vi "LiDAR_UI.vi"() -> ()   [LabVIEW 2020]
doc: "This template is for the Queued Message Handler design pattern.\n\nThe Event Handling Loop generates messages based on user interface actions.\n\nThe Message Handling Loop processes messages generated by the Event Handling Loop, or by other messages. The messages are string values, so new messages can be added easily to the Message Cases case structure in the Message Handling Loop. Each message cluster can also provide an optional value for Message Data, which is a variant that can be converted to whatever message-specific data is required."
uses:
  controls/UI Data.ctl
  support/Message Queue/Enqueue Message (Single).vi
  <vilib>/Instr/_visa.llb/VISA Configure Serial Port (Instr).vi
  <vilib>/Utility/error.llb/Error Cluster From Error Code.vi
  <vilib>/ErrorRing/Error Ring.xnode
  support/Message Queue/Message Queue.lvlib
  support/User Event - Stop/User Event - Stop.lvlib
  <vilib>/Analysis/NI_AALBase.lvlib
panel:
  in  "?":T1(tab)
  out "Waveform Graph":dbl[](graph)
  in  "LASER ON/OFF":bool
  out "Duty Cycle":dbl(slide) scale=0.0..0.001
  in  "Exit":bool
  in  "Pulse Length (ns)":dbl(slide) scale=8.0..100.0
  in  "Rep. Rate (Hz)":dbl(slide) scale=0.0..100.0
  in  "Save Settings\nPLCS":bool
  in  "Load Settings\nPLCS":bool
  out "Power (mW)":dbl(slide) scale=0.0..65.0
  out "Warning":bool
  in  "Calibration Current":dbl
  in  "Driver Voltage":dbl
  in  "Save Settings BFS":bool
  in  "TEC Current Limit (A)":dbl(slide) scale=0.0..1.0
  in  "TEC KI":dbl(slide) scale=0.0..0.04
  in  "TEC KP":dbl(slide) scale=0.0..2.0
  in  "TEC Temperatur":dbl(knob) scale=0.0..70.0
  in  "VREF (V)":dbl(slide) scale=0.0..1.0
  in  "Load Settings BFS":bool
  out "Display (BFS-VRM 03)":string
  in  "Numeric":dbl
  in  "Un/Lock":bool
  out "Display (PLCS-21/LDP-V)":string
  in  "Set Max. Duty Cycle":dbl
  in  "Voltage (mv)":dbl(slide) scale=0.0..5600.0
  in  "Current (mA)":u64(slide) scale=0.0..10.0
  in  "Modes":enum32{"Voltage Mode", "Current Mode"}(radio)
  # "Pulser Parameter"
  # "Toggles"
  # "Warnings"
  # "Driver Parameter"
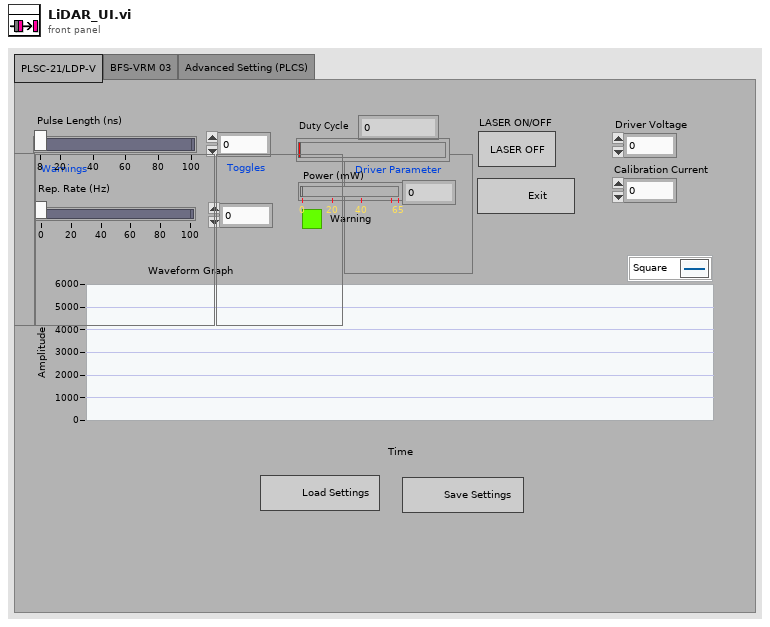
[diagram p1: front panel]
types:
  T1 = enum32{"PLSC-21/LDP-V", "BFS-VRM 03", "Advanced Setting (PLCS)"}
  T2 = typedef "UI Data.ctl" = cluster{"Boolean <Replace Me>":bool, "String <Replace Me>":string, "Numeric <Replace Me>":dbl, "LASER ON/OFF Ref":refnum<vi>, "Do Something Else Ref":refnum<vi>, "Data Display Ref":refnum<vi>, "Exit Button Ref":refnum<vi>}
  T3 = typedef "Message Queue.lvlib/All Message Queues.ctl" = cluster{"UI":refnum<queue>}
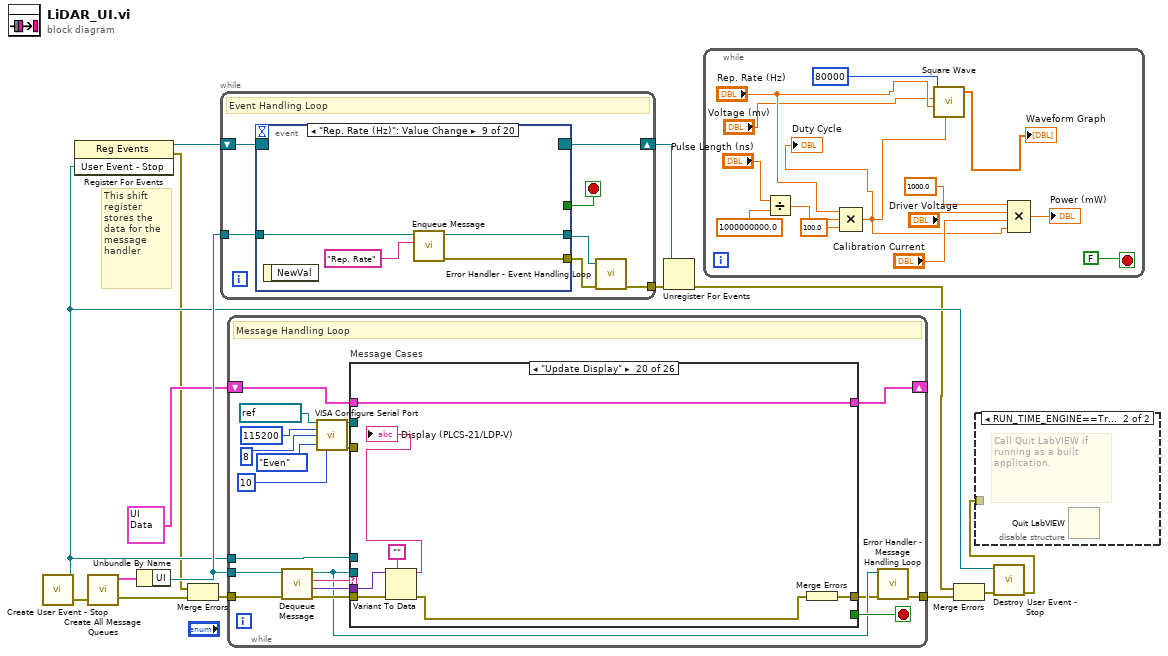
[diagram p0: block diagram]
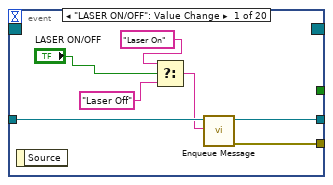
[diagram p3: hidden frame]
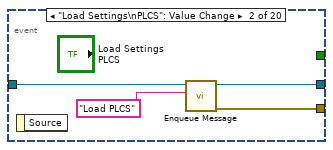
[diagram p4: hidden frame]
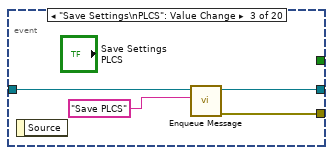
[diagram p5: hidden frame]
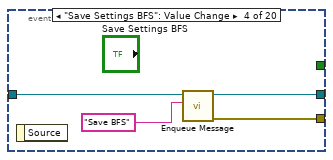
[diagram p6: hidden frame]
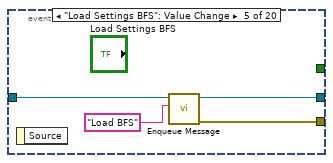
[diagram p7: hidden frame]
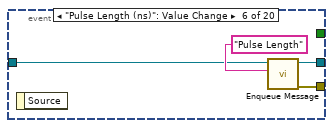
[diagram p8: hidden frame]
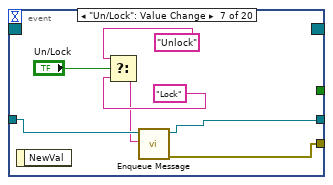
[diagram p9: hidden frame]
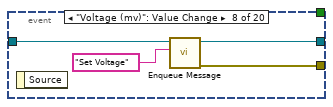
[diagram p10: hidden frame]
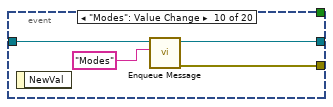
[diagram p11: hidden frame]
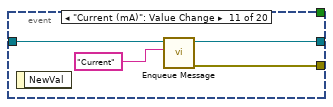
[diagram p12: hidden frame]
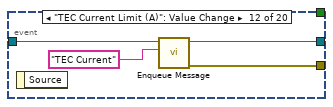
[diagram p13: hidden frame]
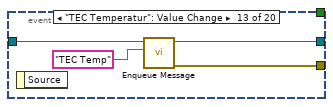
[diagram p14: hidden frame]
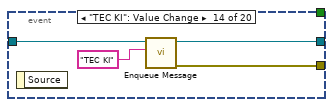
[diagram p15: hidden frame]
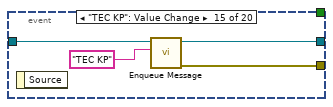
[diagram p16: hidden frame]
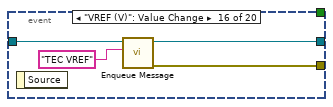
[diagram p17: hidden frame]
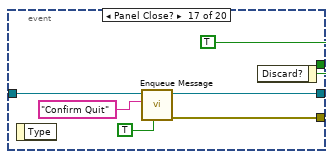
[diagram p18: hidden frame]
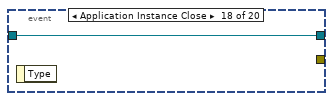
[diagram p19: hidden frame]
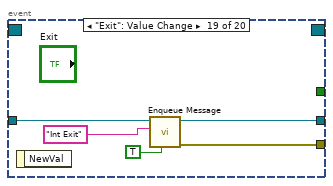
[diagram p20: hidden frame]
diagram:
  # "This shift register stores the data for the message handler"
  n1 = call "Create User Event - Stop.vi"() -> ("error out"=w11:errorcluster, "User Event - Stop"=w5:refnum<user-event>)  [unwired: 10 in]
  n2 = register-events(w5) -> (reference out=w6:refnum<event-registration>, error out=w3:errorcluster)  [unwired: 2 in]
  n3 = call "Create All Message Queues.vi"("error in (no error)"=w11) -> ("error out"=w15:errorcluster, "Message Queues out"=w14:T3)  [unwired: 9 in]
  n4 = Unbundle By Name(w14) -> ("UI"=w12:refnum<queue>)
  n5 = Merge Errors(w3, w15) -> (w4:errorcluster)
  n6 = while {
    tunnel: w12 -> [w22]
    shift-right: [w17] -> w9
    shift-left: w6 -> [w21]
    tunnel: [w19] -> w7
    stop <- w16 stop-if-true
    # "Event Handling Loop"
    n7 = event shown="[8] \"Rep. Rate (Hz)\": Value Change" {
      selector: w21 -> [_ _ _ _ _ _ _ _ _ _ _ _ _ _ _ _ _ _ _ _]
      dyn-events: [_ _ _ _ _ _ _ _ _ _ _ _ _ _ _ _ _ _ _ _] -> w17
      timeout: _ -> [_ _ _ _ _ _ _ _ _ _ _ _ _ _ _ _ _ _ _ _]
      tunnel: [_ _ _ _ _ _ _ _ _ _ _ _ _ _ _ _ _ _ _ TRUE ("Discard?")] -> w16
      tunnel: w22 -> [w29 w33 w37 w40 w44 w46 w54 w60 w64 w68 w72 w76 w80 w84 w88 w92 w97 w99 w104 w107]
      tunnel: [w27 w30 w34 w38 w42 w47 w53 w58 w61 w65 w70 w73 w77 w81 w85 w89 w96 _ w103 _] -> w20
      tunnel: [w28 w32 w36 w41 w45 w48 w55 w59 w63 w67 w71 w75 w79 w83 w87 w91 w95 w99 w102 w107] -> w18
      event "LASER ON/OFF": Value Change {
        n8 = event-data() -> ()  [unwired: 1 in, 1 out]
        n9 = Select(t="Laser On" ("Message"), s="LASER ON/OFF", f="Laser Off" ("Message")) -> (s? t:f=w26:string)
        n10 = call-poly "Enqueue Message.vi"("Message"=w26, "Message Queue"=w29) -> ("error out"=w27:errorcluster, "dup Message Queue"=w28:refnum<queue>)  [unwired: 8 in]
      }
      event "Load Settings\nPLCS": Value Change {
        n11 = event-data() -> ()  [unwired: 1 in, 1 out]
        n12 = call-poly "Enqueue Message.vi"("Message"="Load PLCS", "Message Queue"=w33) -> ("error out"=w30:errorcluster, "dup Message Queue"=w32:refnum<queue>)  [unwired: 8 in]
      }
      event "Save Settings\nPLCS": Value Change {
        n13 = event-data() -> ()  [unwired: 1 in, 1 out]
        n14 = call-poly "Enqueue Message.vi"("Message"="Save PLCS", "Message Queue"=w37) -> ("error out"=w34:errorcluster, "dup Message Queue"=w36:refnum<queue>)  [unwired: 8 in]
      }
      event "Save Settings BFS": Value Change {
        n15 = event-data() -> ()  [unwired: 1 in, 1 out]
        n16 = call-poly "Enqueue Message.vi"("Message"="Save BFS", "Message Queue"=w40) -> ("error out"=w38:errorcluster, "dup Message Queue"=w41:refnum<queue>)  [unwired: 8 in]
      }
      event "Load Settings BFS": Value Change {
        n17 = event-data() -> ()  [unwired: 1 in, 1 out]
        n18 = call-poly "Enqueue Message.vi"("Message"="Load BFS", "Message Queue"=w44) -> ("error out"=w42:errorcluster, "dup Message Queue"=w45:refnum<queue>)  [unwired: 8 in]
      }
      event "Pulse Length (ns)": Value Change {
        n19 = event-data() -> ()  [unwired: 1 in, 1 out]
        n20 = call-poly "Enqueue Message.vi"("Message"="Pulse Length", "Message Queue"=w46) -> ("error out"=w47:errorcluster, "dup Message Queue"=w48:refnum<queue>)  [unwired: 8 in]
      }
      event "Un/Lock": Value Change {
        n21 = event-data() -> ()  [unwired: 1 in, 1 out]
        n22 = Select(t="Unlock", s="Un/Lock", f="Lock") -> (s? t:f=w50:string)
        n23 = call-poly "Enqueue Message.vi"("Message"=w50, "Message Queue"=w54) -> ("error out"=w53:errorcluster, "dup Message Queue"=w55:refnum<queue>)  [unwired: 8 in]
      }
      event "Voltage (mv)": Value Change {
        n24 = event-data() -> ()  [unwired: 1 in, 1 out]
        n25 = call-poly "Enqueue Message.vi"("Message"="Set Voltage", "Message Queue"=w60) -> ("error out"=w58:errorcluster, "dup Message Queue"=w59:refnum<queue>)  [unwired: 8 in]
      }
      event "Rep. Rate (Hz)": Value Change {
        n26 = event-data() -> ()  [unwired: 1 in, 1 out]
        n27 = call-poly "Enqueue Message.vi"("Message"="Rep. Rate", "Message Queue"=w64) -> ("error out"=w61:errorcluster, "dup Message Queue"=w63:refnum<queue>)  [unwired: 8 in]
      }
      event "Modes": Value Change {
        n28 = event-data() -> ()  [unwired: 1 in, 1 out]
        n29 = call-poly "Enqueue Message.vi"("Message"="Modes", "Message Queue"=w68) -> ("error out"=w65:errorcluster, "dup Message Queue"=w67:refnum<queue>)  [unwired: 8 in]
      }
      event "Current (mA)": Value Change {
        n30 = event-data() -> ()  [unwired: 1 in, 1 out]
        n31 = call-poly "Enqueue Message.vi"("Message"="Current", "Message Queue"=w72) -> ("error out"=w70:errorcluster, "dup Message Queue"=w71:refnum<queue>)  [unwired: 8 in]
      }
      event "TEC Current Limit (A)": Value Change {
        n32 = event-data() -> ()  [unwired: 1 in, 1 out]
        n33 = call-poly "Enqueue Message.vi"("Message"="TEC Current", "Message Queue"=w76) -> ("error out"=w73:errorcluster, "dup Message Queue"=w75:refnum<queue>)  [unwired: 8 in]
      }
      event "TEC Temperatur": Value Change {
        n34 = event-data() -> ()  [unwired: 1 in, 1 out]
        n35 = call-poly "Enqueue Message.vi"("Message"="TEC Temp", "Message Queue"=w80) -> ("error out"=w77:errorcluster, "dup Message Queue"=w79:refnum<queue>)  [unwired: 8 in]
      }
      event "TEC KI": Value Change {
        n36 = event-data() -> ()  [unwired: 1 in, 1 out]
        n37 = call-poly "Enqueue Message.vi"("Message"="TEC KI", "Message Queue"=w84) -> ("error out"=w81:errorcluster, "dup Message Queue"=w83:refnum<queue>)  [unwired: 8 in]
      }
      event "TEC KP": Value Change {
        n38 = event-data() -> ()  [unwired: 1 in, 1 out]
        n39 = call-poly "Enqueue Message.vi"("Message"="TEC KP", "Message Queue"=w88) -> ("error out"=w85:errorcluster, "dup Message Queue"=w87:refnum<queue>)  [unwired: 8 in]
      }
      event "VREF (V)": Value Change {
        n40 = event-data() -> ()  [unwired: 1 in, 1 out]
        n41 = call-poly "Enqueue Message.vi"("Message"="TEC VREF", "Message Queue"=w92) -> ("error out"=w89:errorcluster, "dup Message Queue"=w91:refnum<queue>)  [unwired: 8 in]
      }
      event Panel Close? {
        n42 = event-data() -> ()  [unwired: 1 in, 1 out]
        n43 = call-poly "Enqueue Message.vi"("Priority Message? (F)"=TRUE, "Message"="Confirm Quit", "Message Queue"=w97) -> ("error out"=w96:errorcluster, "dup Message Queue"=w95:refnum<queue>)  [unwired: 7 in]
        n44 = event-data("Discard?"=TRUE) -> ()  [unwired: 1 in, 1 out]
      }
      event Application Instance Close {
        n45 = event-data() -> ()  [unwired: 1 in, 1 out]
      }
      event "Exit": Value Change {
        n46 = event-data() -> ()  [unwired: 1 in, 1 out]
        n47 = call-poly "Enqueue Message.vi"("Priority Message? (F)"=TRUE, "Message"="Int Exit", "Message Queue"=w104) -> ("error out"=w103:errorcluster, "dup Message Queue"=w102:refnum<queue>)  [unwired: 7 in]
      }
      event User Event {
        n48 = event-data() -> ()  [unwired: 1 in, 1 out]
        n49 = local write "Display (PLCS-21/LDP-V)"("\"Exit\" button pressed/COM Released" ("VI Stopped")) -> ()
      }
    }
    n50 = call "Error Handler - Event Handling Loop.vi"("error in (no error)"=w20, "Message Queue"=w18) -> ("dup error in"=w19:errorcluster)  [unwired: 8 in, 1 out]
  }
  n51 = while {
    tunnel: w12 -> [w118]
    shift-right: [w125] -> _
    shift-left: T2 {"Boolean <Replace Me>"=FALSE, "String <Replace Me>"="", "Numeric <Replace Me>"=0.0, "LASER ON/OFF Ref"=refnum, "Do Something Else Ref"=refnum, "Data Display Ref"=refnum, "Exit Button Ref"=refnum} ("Data Cluster") -> [w126]
    tunnel: w5 -> [w123]
    tunnel: w4 -> [w122]
    tunnel: [w116] -> w13
    stop <- w124 stop-if-true
    # "Message Handling Loop"
    n52 = call "Dequeue Message.vi"("error in (no error)"=w122, "Message Queue"=w118) -> ("error out"=w121:errorcluster, "Message Data"=w119:variant, "Message"=w120:string, "dup Message Queue"=w117:refnum<queue>)  [unwired: 6 in]
    n53 = call-poly "VISA Configure Serial Port"("VISA resource name"=refnum<visa-resource-name> "COM4", "baud rate (9600)"=u32 115200, "data bits (8)"=u16 8, "parity (0:none)"=enum16{"None", "Odd", "Even", "Mark", "Space"}."Even", "stop bits (10: 1 bit)"=u16 10) -> ("VISA resource name out"=w109:refnum<visa-resource-name>, "error out"=w108:errorcluster)  [unwired: 9 in]
    n54 = case "Message Cases" shown="\"Update Display\"" w120 {
      selector: w120 -> [_ _ _ _ _ _ _ _ _ _ _ _ _ _ _ _ _ _ _ _ _ _ _ _ _ w431]
      tunnel: w117 -> [w134 w153 w168 w186 w205 w211 w236 w254 w272 w290 w308 w319 w330 _ _ _ _ _ _ _ _ _ w401 w408 w430 _]
      tunnel: w121 -> [w135 w154 w170 w188 w207 w213 w238 w256 w274 w292 w310 w321 w332 w342 w345 w353 w361 w369 w377 w383 w389 w398 w405 w409 w423 _]
      tunnel: [w133 w156 w169 w187 w206 w212 w237 w255 w273 w291 w309 w322 w333 w342 w345 w353 w361 w369 w377 w384 w390 w392 w403 w413 w426 w432] -> w115
      tunnel: w126 -> [w140 w143 w173 w179 w210 w222 w240 w258 w276 w294 w312 w323 w334 w341 w344 w352 w360 w368 w376 w378 w391 w397 w404 w414 w429 w433]
      tunnel: [w139 w143 w173 w179 w210 w222 w240 w258 w276 w294 w312 w323 w334 w341 w344 w352 w360 w368 w376 w378 w391 w397 w404 w414 w429 w433] -> w125
      tunnel: [_ _ _ _ _ _ _ _ _ _ _ _ _ _ _ _ _ _ _ _ _ _ _ _ TRUE _] -> w124
      tunnel: w119 -> [_ _ _ _ _ _ _ _ _ _ _ _ _ _ _ _ _ _ _ w382 w388 w396 _ _ w420 _]
      tunnel: w123 -> [_ _ _ _ _ _ _ _ _ _ _ _ _ _ _ _ _ _ _ _ _ _ _ _ w425 _]
      tunnel: w109 -> [_ w161 w172 w194 w204 w221 _ _ _ _ _ w317 w326 _ _ _ _ _ _ _ _ _ _ _ w419 _]
      tunnel: w108 -> [_ w160 w171 w193 w203 w220 _ _ _ _ _ w316 w325 _ _ _ _ _ _ _ _ _ _ _ w418 _]
      frame "Initialize" {
        w132 = "Laser Off" ("Initial Message")
        # "Initialize - All initialization work should take place in this message, since other loops can potentially enqueue messages that execute immediately after this one."
        n55 = control-ref of="Exit"() -> (w137:refnum<vi>)
        n56 = control-ref of="Display (PLCS-21/LDP-V)"() -> (w138:refnum<vi>)
        n57 = control-ref of="LASER ON/OFF"() -> (w136:refnum<vi>)
        n58 = property on="Pulse Length (ns)" class="Slide (strict)"("Scale.Maximum"="Numeric") -> ()  [unwired: 2 in, 2 out]
        n59 = local write "Warning"(FALSE) -> ()
        n60 = call-poly "Enqueue Message.vi"("error in (no error)"=w135, "Message"=w132, "Message Queue"=w134) -> ("error out"=w133:errorcluster)  [unwired: 7 in, 1 out]
        n61 = Bundle By Name(cluster=w140, "LASER ON/OFF Ref"=w136, "Data Display Ref"=w138, "Exit Button Ref"=w137, "String <Replace Me>"=w132) -> (w139:T2)
        n62 = call "Convert to Dynamic Data"("Array"=dbl[] [] ("History Data")) -> ("Dynamic Data Type"=w129:dynamicdata)  [unwired: 3 in]
        n63 = call "Convert from Dynamic Data"("Dynamic Data Type"=w129) -> ("Array"=w127:dbl[])  [unwired: 3 in]
        n64 = local write "Waveform Graph"(w127) -> ()
      }
      frame "Pulse Length" {
        n65 = local read "Pulse Length (ns)"() -> (w155:dbl)
        n66 = local read "Duty Cycle"() -> (w150:dbl)
        n67 = Concatenate Strings("Laseroff" ("Message"), "\r") -> (w144:string)
        n68 = Number To Decimal String(number=w155) -> (decimal integer string=w158:string)  [unwired: 1 in]
        n69 = Greater?(x=w150, y="Set Max. Duty Cycle") -> (0:w141:bool)
        "Warning" <- w141
        n70 = Select(t="Laser Off" ("Message"), s=w141, f="Update Display" ("Message")) -> (s? t:f=w149:string)
        n71 = Concatenate Strings("spulse ", w158, "\r") -> (w152:string)
        n72 = Select(t=w152, s=w141, f=w144) -> (s? t:f=w151:string)
        n73 = VISA Write(VISA resource name=w161, write buffer=w151, error in (no error)=w160) -> ()  [unwired: 3 out]
        n74 = call-poly "Enqueue Message.vi"("error in (no error)"=w154, "Message Data"=w151, "Message"=w149, "Message Queue"=w153) -> ("error out"=w156:errorcluster)  [unwired: 6 in, 1 out]
      }
      frame "Set Voltage" {
        n75 = local read "Voltage (mv)"() -> (w162:dbl)
        n76 = Number To Decimal String(number=w162) -> (decimal integer string=w165:string)  [unwired: 1 in]
        n77 = Concatenate Strings("svoltage  ", w165, "\r") -> (w163:string)
        n78 = VISA Write(VISA resource name=w172, write buffer=w163, error in (no error)=w171) -> ()  [unwired: 3 out]
        n79 = call-poly "Enqueue Message.vi"("error in (no error)"=w170, "Message Data"=w163, "Message"="Update Display", "Message Queue"=w168) -> ("error out"=w169:errorcluster)  [unwired: 6 in, 1 out]
      }
      frame "Rep. Rate" {
        n80 = local read "Set Max. Duty Cycle"() -> (w175:dbl)
        n81 = local read "Rep. Rate (Hz)"() -> (w189:dbl)
        n82 = local read "Duty Cycle"() -> (w180:dbl)
        n83 = Concatenate Strings("laseroff ", "\r") -> (w182:string)
        n84 = Number To Decimal String(number=w189) -> (decimal integer string=w191:string)  [unwired: 1 in]
        n85 = Greater?(x=w180, y=w175) -> (0:w174:bool)
        n86 = Select(t="Laser Off" ("Message"), s=w174, f="Update Display" ("Message")) -> (s? t:f=w177:string)
        n87 = Concatenate Strings("sreprate  ", w191, "\r") -> (w185:string)
        n88 = Select(t=w185, s=w174, f=w182) -> (s? t:f=w181:string)
        n89 = VISA Write(VISA resource name=w194, write buffer=w181, error in (no error)=w193) -> ()  [unwired: 3 out]
        n90 = local write "Warning"(w174) -> ()
        n91 = call-poly "Enqueue Message.vi"("error in (no error)"=w188, "Message Data"=w181, "Message"=w177, "Message Queue"=w186) -> ("error out"=w187:errorcluster)  [unwired: 6 in, 1 out]
      }
      frame "Modes" {
        n92 = Equal To 0?(x="Modes") -> (x = 0?=w209:bool)
        n93 = Select(t=1, s=w209, f=2) -> (s? t:f=w200:i32)
        n94 = Number To Decimal String(number=w200) -> (decimal integer string=w199:string)  [unwired: 1 in]
        n95 = Concatenate Strings("smode ", w199, "\r") -> (w195:string)
        n96 = VISA Write(VISA resource name=w204, write buffer=w195, error in (no error)=w203) -> ()  [unwired: 3 out]
        n97 = call-poly "Enqueue Message.vi"("error in (no error)"=w207, "Message Data"=w195, "Message"="Update Display", "Message Queue"=w205) -> ("error out"=w206:errorcluster)  [unwired: 6 in, 1 out]
      }
      frame "Current" {
        n98 = Number To Decimal String(number="Current (mA)") -> (decimal integer string=w219:string)  [unwired: 1 in]
        n99 = Concatenate Strings("scurrent  ", w219, "\r") -> (w215:string)
        n100 = VISA Write(VISA resource name=w221, write buffer=w215, error in (no error)=w220) -> ()  [unwired: 3 out]
        n101 = call-poly "Enqueue Message.vi"("error in (no error)"=w213, "Message Data"=w215, "Message"="Update Display", "Message Queue"=w211) -> ("error out"=w212:errorcluster)  [unwired: 6 in, 1 out]
      }
      frame "TEC Current" {
        n102 = local read "TEC Current Limit (A)"() -> (w235:dbl)
        n103 = call-poly "VISA Configure Serial Port"("VISA resource name"=refnum<visa-resource-name> "COM3", "baud rate (9600)"=u32 115200, "data bits (8)"=u16 8, "parity (0:none)"=enum16{"None", "Odd", "Even", "Mark", "Space"}."Even", "stop bits (10: 1 bit)"=u16 10) -> ("VISA resource name out"=w224:refnum<visa-resource-name>, "error out"=w223:errorcluster)  [unwired: 9 in]
        n104 = Number To Fractional String(number=w235, precision (6)=2) -> (F-format string=w234:string)  [unwired: 2 in]
        n105 = Concatenate Strings("simax  ", w234, "\r") -> (w230:string)
        n106 = VISA Write(VISA resource name=w224, write buffer=w230, error in (no error)=w223) -> ()  [unwired: 3 out]
        n107 = call-poly "Enqueue Message.vi"("error in (no error)"=w238, "Message Data"=w230, "Message"="Display 2", "Message Queue"=w236) -> ("error out"=w237:errorcluster)  [unwired: 6 in, 1 out]
      }
      frame "TEC Temp" {
        w250 = "stsoll  "  # stsoll
        n108 = local read "TEC Temperatur"() -> (w253:dbl)
        n109 = call-poly "VISA Configure Serial Port"("VISA resource name"=refnum<visa-resource-name> "COM3", "baud rate (9600)"=u32 115200, "data bits (8)"=u16 8, "parity (0:none)"=enum16{"None", "Odd", "Even", "Mark", "Space"}."Even", "stop bits (10: 1 bit)"=u16 10) -> ("VISA resource name out"=w242:refnum<visa-resource-name>, "error out"=w241:errorcluster)  [unwired: 9 in]
        n110 = Number To Fractional String(number=w253, precision (6)=0) -> (F-format string=w252:string)  [unwired: 2 in]
        n111 = Concatenate Strings(w250, w252, "\r") -> (w248:string)
        n112 = VISA Write(VISA resource name=w242, write buffer=w248, error in (no error)=w241) -> ()  [unwired: 3 out]
        n113 = call-poly "Enqueue Message.vi"("error in (no error)"=w256, "Message Data"=w248, "Message"="Display 2", "Message Queue"=w254) -> ("error out"=w255:errorcluster)  [unwired: 6 in, 1 out]
      }
      frame "TEC KI" {
        w268 = "ski  "  # ski
        n114 = local read "TEC KI"() -> (w271:dbl)
        n115 = call-poly "VISA Configure Serial Port"("VISA resource name"=refnum<visa-resource-name> "COM3", "baud rate (9600)"=u32 115200, "data bits (8)"=u16 8, "parity (0:none)"=enum16{"None", "Odd", "Even", "Mark", "Space"}."Even", "stop bits (10: 1 bit)"=u16 10) -> ("VISA resource name out"=w260:refnum<visa-resource-name>, "error out"=w259:errorcluster)  [unwired: 9 in]
        n116 = Number To Fractional String(number=w271, precision (6)=2) -> (F-format string=w270:string)  [unwired: 2 in]
        n117 = Concatenate Strings(w268, w270, "\r") -> (w266:string)
        n118 = VISA Write(VISA resource name=w260, write buffer=w266, error in (no error)=w259) -> ()  [unwired: 3 out]
        n119 = call-poly "Enqueue Message.vi"("error in (no error)"=w274, "Message Data"=w266, "Message"="Display 2", "Message Queue"=w272) -> ("error out"=w273:errorcluster)  [unwired: 6 in, 1 out]
      }
      frame "TEC KP" {
        w286 = "skp  "  # skp
        n120 = local read "TEC KP"() -> (w289:dbl)
        n121 = call-poly "VISA Configure Serial Port"("VISA resource name"=refnum<visa-resource-name> "COM3", "baud rate (9600)"=u32 115200, "data bits (8)"=u16 8, "parity (0:none)"=enum16{"None", "Odd", "Even", "Mark", "Space"}."Even", "stop bits (10: 1 bit)"=u16 10) -> ("VISA resource name out"=w278:refnum<visa-resource-name>, "error out"=w277:errorcluster)  [unwired: 9 in]
        n122 = Number To Fractional String(number=w289, precision (6)=2) -> (F-format string=w288:string)  [unwired: 2 in]
        n123 = Concatenate Strings(w286, w288, "\r") -> (w284:string)
        n124 = VISA Write(VISA resource name=w278, write buffer=w284, error in (no error)=w277) -> ()  [unwired: 3 out]
        n125 = call-poly "Enqueue Message.vi"("error in (no error)"=w292, "Message Data"=w284, "Message"="Display 2", "Message Queue"=w290) -> ("error out"=w291:errorcluster)  [unwired: 6 in, 1 out]
      }
      frame "TEC VREF" {
        w304 = "svref "  # svref
        n126 = local read "VREF (V)"() -> (w307:dbl)
        n127 = call-poly "VISA Configure Serial Port"("VISA resource name"=refnum<visa-resource-name> "COM3", "baud rate (9600)"=u32 115200, "data bits (8)"=u16 8, "parity (0:none)"=enum16{"None", "Odd", "Even", "Mark", "Space"}."Even", "stop bits (10: 1 bit)"=u16 10) -> ("VISA resource name out"=w296:refnum<visa-resource-name>, "error out"=w295:errorcluster)  [unwired: 9 in]
        n128 = Number To Fractional String(number=w307, precision (6)=2) -> (F-format string=w306:string)  [unwired: 2 in]
        n129 = Concatenate Strings(w304, w306, "\r") -> (w302:string)
        n130 = VISA Write(VISA resource name=w296, write buffer=w302, error in (no error)=w295) -> ()  [unwired: 3 out]
        n131 = call-poly "Enqueue Message.vi"("error in (no error)"=w310, "Message Data"=w302, "Message"="Display 2", "Message Queue"=w308) -> ("error out"=w309:errorcluster)  [unwired: 6 in, 1 out]
      }
      frame "Laser On" {
        # "Send string to \"Update Display\" message"
        # "Something - Replace this message with functionality for your own application."
        n132 = Concatenate Strings("laseron", "\r") -> (w313:string)
        n133 = VISA Write(VISA resource name=w317, write buffer=w313, error in (no error)=w316) -> ()  [unwired: 3 out]
        n134 = call-poly "Enqueue Message.vi"("error in (no error)"=w321, "Message Data"=w313, "Message"="Update Display", "Message Queue"=w319) -> ("error out"=w320:errorcluster)  [unwired: 6 in, 1 out]
        n135 = Merge Errors(w320) -> (w322:errorcluster)
      }
      frame "Laser Off" {
        # "Something Else - Replace this message with functionality for your own application."
        n136 = Concatenate Strings("laseroff", "\r") -> (w324:string)
        n137 = VISA Write(VISA resource name=w326, write buffer=w324, error in (no error)=w325) -> ()  [unwired: 3 out]
        n138 = call-poly "Enqueue Message.vi"("error in (no error)"=w332, "Message Data"=w324, "Message"="Update Display", "Message Queue"=w330) -> ("error out"=w331:errorcluster)  [unwired: 6 in, 1 out]
        n139 = Merge Errors(w331) -> (w333:errorcluster)
      }
      frame "Unlock" {
        # "Unlock safe limit if pawwsord\nmatch"
        # "Compare password"
        n140 = call "Request Password"() -> ("Password"=w340:string)  [unwired: 17 in, 2 out]
        n141 = Equal?(x=w340, y="abc") -> (x = y?=w338:bool)
        n142 = Select(t=enum16{"Enabled", "Disabled"}."Enabled", s=w338, f=enum16{"Enabled", "Disabled"}."Disabled") -> (s? t:f=w335:enum16{"Enabled", "Disabled"})
        n143 = property on="Set Max. Duty Cycle" class="DigNum (strict)"("DisabledEnum"=w335) -> ()  [unwired: 2 in, 2 out]
      }
      frame "Lock" {
        # "Disable Changing safe limit"
        n144 = property on="Set Max. Duty Cycle" class="DigNum (strict)"("DisabledEnum"=enum16{"Enabled", "Disabled"}."Disabled") -> ()  [unwired: 2 in, 2 out]
      }
      frame "Save BFS" {
        n145 = Merge Signals("TEC Temperatur", "VREF (V)", "TEC KI", "TEC KP", "TEC Current Limit (A)") -> (w351:dynamicdata)
        n146 = call "Write To Measurement File"("Signals"=w351) -> ()  [unwired: 16 in, 3 out]
      }
      frame "Save PLCS" {
        n147 = local read "Pulse Length (ns)"() -> (w355:dbl)
        n148 = local read "Rep. Rate (Hz)"() -> (w358:dbl)
        n149 = local read "Voltage (mv)"() -> (w356:dbl)
        n150 = local read "Set Max. Duty Cycle"() -> (w354:dbl)
        n151 = local read "Current (mA)"() -> (w357:u64)
        n152 = Merge Signals(w358, w356, w355, w357, w354) -> (w359:dynamicdata)
        n153 = call "Write To Measurement File2"("Signals"=w359) -> ()  [unwired: 16 in, 3 out]
      }
      frame "Load BFS" {
        n154 = call "Read From Measurement File"() -> ("Signals"=w362:dynamicdata)  [unwired: 6 in, 5 out]
        n155 = Split Signals(w362) -> (w363:dynamicdata, w364:dynamicdata, w367:dynamicdata, w365:dynamicdata, w366:dynamicdata)  [unwired: 5 in]
        n156 = property on="TEC Current Limit (A)" class="Slide (strict)"("Value"=w363) -> ()  [unwired: 2 in, 2 out]
        n157 = property on="TEC KP" class="Slide (strict)"("Value"=w364) -> ()  [unwired: 2 in, 2 out]
        n158 = property on="TEC KI" class="Slide (strict)"("Value"=w367) -> ()  [unwired: 2 in, 2 out]
        n159 = property on="VREF (V)" class="Slide (strict)"("Value"=w365) -> ()  [unwired: 2 in, 2 out]
        n160 = property on="TEC Temperatur" class="Knob (strict)"("Value"=w366) -> ()  [unwired: 2 in, 2 out]
      }
      frame "Load PLCS" {
        n161 = call "Read From Measurement File2"() -> ("Signals"=w375:dynamicdata)  [unwired: 6 in, 5 out]
        n162 = Split Signals(w375) -> (w374:dynamicdata, w373:dynamicdata, w372:dynamicdata, w371:dynamicdata, w370:dynamicdata)  [unwired: 5 in]
        n163 = property on="Rep. Rate (Hz)" class="Slide (strict)"("Value"=w374) -> ()  [unwired: 2 in, 2 out]
        n164 = property on="Current (mA)" class="Slide (strict)"("Value"=w371) -> ()  [unwired: 2 in, 2 out]
        n165 = property on="Pulse Length (ns)" class="Slide (strict)"("Value"=w373) -> ()  [unwired: 2 in, 2 out]
        n166 = property on="Voltage (mv)" class="Slide (strict)"("Value"=w372) -> ()  [unwired: 2 in, 2 out]
        n167 = property on="Set Max. Duty Cycle" class="DigNum (strict)"("Value"=w370) -> ()  [unwired: 2 in, 2 out]
      }
      frame "Update Display" {
        # "Update Display - Convert the message data to a string to display in the Data Display indicator."
        n168 = Variant To Data(error in=w383, type="", Variant=w382) -> (data=→"Display (PLCS-21/LDP-V)":string, error out=w379:errorcluster)
        n169 = Merge Errors(w379) -> (w384:errorcluster)
      }
      frame "Display 2" {
        # "#CodeRecommended - If you wish to decouple the Message Handling Loop from your user interface, consider creating User Events (like the \"Stop\" event in this VI) to message the Event Handling Loop whenever the user interface needs updating."
        # "Update Display - Convert the message data to a string to display in the Data Display indicator."
        n170 = Variant To Data(error in=w389, type="", Variant=w388) -> (data=→"Display (BFS-VRM 03)":string, error out=w386:errorcluster)
        n171 = Merge Errors(w386) -> (w390:errorcluster)
      }
      frame "Error" {
        # "#CodeRecommended - If you ever change the name of this \"Error\" message, you'll need to update the name in the Check Loop Error.vi as well."
        # "#CodeRecommended - Consider creating a system for logging errors in some way. These errors are for notification purposes only. Handling of specific errors should be performed in the message frames that generated the error."
        # "Error - Display an error dialog. This message is sent by the \"Error Handler\" VIs at the end of other loops in this application."
        n172 = Variant To Data(error in=w398, type=errorcluster {"status"=FALSE, "code"=0, "source"=""} ("error constant"), Variant=w396) -> (data=w394:errorcluster, error out=w393:errorcluster)
        n173 = call <vilib>:"Simple Error Handler.vi"("error in (no error)"=w394) -> ()  [unwired: 4 in, 5 out]
        n174 = Merge Errors(w393) -> (w392:errorcluster)
      }
      frame "Confirm Quit" {
        # "#CodeNeeded - If you want to provide an \"Are you sure\" dialog (or some other notification) before the application exits, place that code here. This message is typically sent from a Panel Close? event."
        # "Confirm Quit - Message that can confirm whether or not the user wants to exit the application."
        n175 = call-poly "Enqueue Message.vi"("Priority Message? (F)"=TRUE, "error in (no error)"=w405, "Message"="Exit", "Message Queue"=w401) -> ("error out"=w402:errorcluster)  [unwired: 6 in, 1 out]
        n176 = Merge Errors(w402) -> (w403:errorcluster)
      }
      frame "Int Exit" {
        # "Duplicate this frame when creating new messages.  Change this comment in the duplicated frame to describe this message."
        n177 = call-poly "Enqueue Message.vi"("error in (no error)"=w409, "Message"="Laser Off", "Message Queue"=w408) -> ("error out"=w410:errorcluster, "dup Message Queue"=w412:refnum<queue>)  [unwired: 7 in]
        n178 = call-poly "Enqueue Message.vi"("error in (no error)"=w410, "Message"="Exit", "Message Queue"=w412) -> ("error out"=w411:errorcluster)  [unwired: 7 in, 1 out]
        n179 = Merge Errors(w411) -> (w413:errorcluster)
      }
      frame "Exit" {
        # "Stop the VI"
        # "Release the message queue reference"
        # "Exit - Exit the application."
        n180 = Variant To Data(type=errorcluster {"status"=FALSE, "code"=0, "source"=""} ("error constant"), Variant=w420) -> (data=w421:errorcluster)  [unwired: 1 in, 1 out]
        n181 = VISA Close(VISA resource name=w419, error in (no error)=w418) -> ()  [unwired: 1 out]
        n182 = call <vilib>:"Simple Error Handler.vi"("error in (no error)"=w421) -> ()  [unwired: 4 in, 5 out]
        n183 = call "Fire User Event - Stop.vi"("User Event - Stop"=w425) -> ("error out"=w424:errorcluster)  [unwired: 10 in]
        n184 = Release Queue(queue=w430, error in (no error)=w423) -> (error out=w427:errorcluster)  [unwired: 1 in, 2 out]
        n185 = call "Convert to Dynamic Data2"("Array"=dbl[] [] ("History Data")) -> ("Dynamic Data Type"=w416:dynamicdata)  [unwired: 3 in]
        n186 = call "Convert from Dynamic Data2"("Dynamic Data Type"=w416) -> ("Array"=w415:dbl[])  [unwired: 3 in]
        n187 = local write "Waveform Graph"(w415) -> ()
        n188 = Merge Errors(w424, w427) -> (w426:errorcluster)
      }
      frame Default {
        # "'Default' case only runs if there is a message that isn't defined in any of the other cases.  Output a programming error."
        n189 = xnode "Error Ring"("parameter 0"=w431) -> ("error out"=w432:errorcluster)
      }
    }
    n190 = call "Error Handler - Message Handling Loop.vi"("error in (no error)"=w115, "Message Queue"=w117) -> ("dup error in"=w116:errorcluster)  [unwired: 8 in, 1 out]
  }
  n191 = Unregister For Events(event registration refnum=w9, error in=w7) -> (error out=w1:errorcluster)
  n192 = while {
    stop <- FALSE stop-if-true
    n193 = Divide(x="Pulse Length (ns)", y=1000000000.0) -> (x/y=w453:dbl)
    n194 = Compound Arithmetic op=MULTIPLY("Rep. Rate (Hz)", w453, 100.0) -> (w443:dbl)
    "Duty Cycle" <- w443
    n195 = call <vilib>:"Square Wave.vi"("samples"=80000, "amplitude"="Voltage (mv)", "frequency"="Rep. Rate (Hz)", "duty cycle (%)"=w443) -> ("square wave"=→"Waveform Graph":dbl[])  [unwired: 2 in, 2 out]
    n196 = Compound Arithmetic op=MULTIPLY(1000.0, "Driver Voltage", "Calibration Current", w443) -> (→"Power (mW)":dbl)
  }
  n197 = Merge Errors(w1, w13) -> (w10:errorcluster)
  n198 = call "Destroy User Event - Stop.vi"("error in (no error)"=w10, "User Event - Stop"=w5) -> ("error out"=w2:errorcluster)  [unwired: 9 in]
  n199 = disable-structure shown="RUN_TIME_ENGINE==True" {
    disable-tunnel: w2 -> [_ _]
    frame condition #0 (active) {
    }
    frame condition #1 {
      # "Call Quit LabVIEW if running as a built application."
      n200 = Quit LabVIEW() -> ()  [unwired: 1 in]
    }
  }
